vi "SaveConfig.vi"(8 "error in (no error)":errorcluster, 11 "DAQ_Module in":refnum<class "DAQ_Module.lvclass">) -> (0 "error out":errorcluster, 3 "DAQ_Module out":refnum<class "DAQ_Module.lvclass">)   [LabVIEW 2025, in "DAQ_Module.lvlib" / "DAQ_Module.lvclass"]
uses:
  DAQ_Module.lvclass
  DAQ_Module.lvclass/DAQ_Module.ctl
  Read TaskConfig.vi
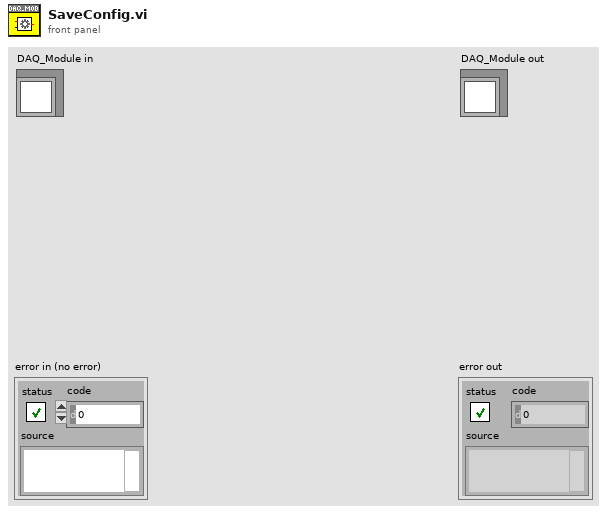
[diagram p1: front panel]
types:
  T1 = typedef "DAQ_Module.lvlib/DAQ_Module.lvclass/DAQ_Config.ctl" = map{string, T2}
  T2 = typedef "DAQ_Module.lvlib/DAQ_Module.lvclass/DAQ_Task_Config.ctl" = cluster{"Drive":T3, "TaskType":T4, "PhysicalChannels":string, "SampleRateConfiguration":T5, "ChannelConfig":map{string, cluster{"Name":string, "Config":string}}, "Enable":bool, "Original":bool}
  T3 = typedef "DAQ_Module.lvlib/DAQ_Module.lvclass/DAQ_HW_Type.ctl" = enum16{"NI_DAQmx", "Simulated_DAQ"}
  T4 = typedef "DAQ_Module.lvlib/DAQ_Module.lvclass/DAQ_Task_Type.ctl" = enum16{"AI", "Linear", "Angular", "AO"}
  T5 = typedef "DAQ_Module.lvlib/DAQ_Module.lvclass/DAQ_SampleRateConfig.ctl" = cluster{"SampleRate":dbl, "SamplesPerChannel":u32, "SamplesPerRead":i32, "SampleMode":i32, "Clock Source":string}
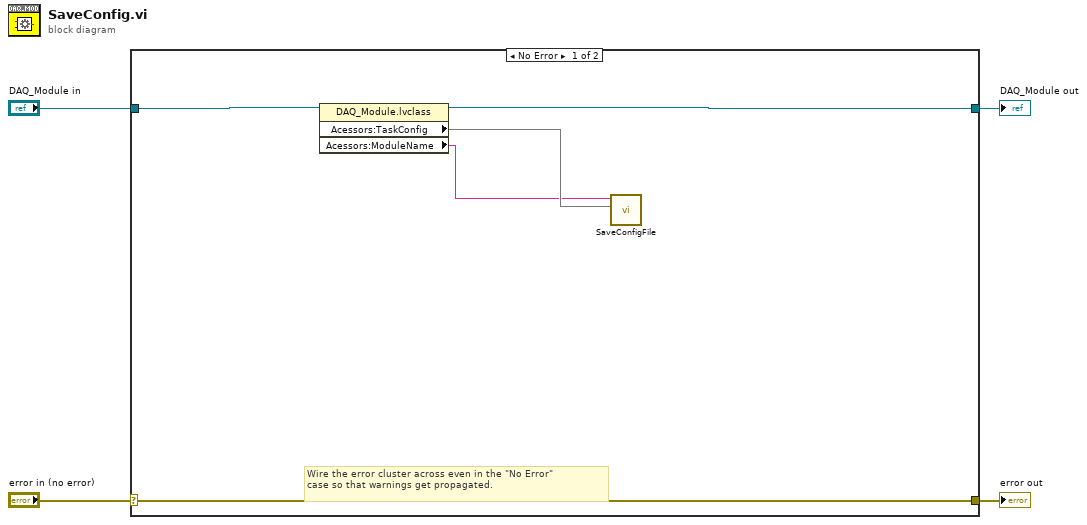
[diagram p0: block diagram]
diagram:
  n1 = case shown="No Error" "error in (no error)" {
    selector: "error in (no error)" -> [w8 w11]
    tunnel: [w8 w11] -> w3
    tunnel: [w7 w10] -> w1
    tunnel: "DAQ_Module in" -> [w9 w10]
    frame No Error {
      # "Wire the error cluster across even in the \"No Error\"\ncase so that warnings get propagated."
      n2 = property class="DAQ_Module.lvclass"(reference=w9) -> (reference out=w7:refnum<class "DAQ_Module.lvclass">, "Acessors:TaskConfig"=w6:T1, "Acessors:ModuleName"=w5:string)  [unwired: 1 in, 1 out]
      n3 = call "SaveConfigFile.vi"("Map"=w6, "Model Name"=w5) -> ()  [unwired: 9 in, 1 out]
    }
    frame Error {
    }
  }
  "error out" <- w3
  "DAQ_Module out" <- w1
